vi "AlliGator Compute Valid Pixels Array.vi"(7 "Optional Rectangle":i32[](array[numeric]), 8 "error in (no error)":errorcluster, 10 "Pixel Counts Constraints":T1 {"High Count Pixels Rejection Options"."High Percentile" min=0.0 max=100.0; "Low Count Pixels Rejection Options"."Low Percentile" min=0.0 max=100.0}, 11 "Sum Image":T4) -> (0 "error out":errorcluster, 1 "CPU (s)":dbl, 2 "[[Valid Pixel (1,NaN)]] VxH Array":sgl[][](array[numeric]), 3 "[[Valid Pixel]] VxH Array":bool[][](array[boolean]), 4 "Message":string)   [LabVIEW 2021, in "AlliGator Phasor Plot.lvlib"]
doc: "Computes a boolean array specifying whether each pixel is valid (verifies all user-defined constraints)."
uses:
  AlliGator Phasor Plot.lvlib
  <vilib>/vision/Image Controls.llb/IMAQ Image.ctl
  AlliGator Pixel Counts Constraints.ctl
  AlliGator High Count Pixels Rejection Options.ctl
  AlliGator Low Count Pixels Rejection Options.ctl
  AlliGator Settings List.ctl
  <vilib>/vision/EDVR.llb/IMAQ ImageToEDVR 2D SGL.vi
  Variant/Variant to Data/Variant to Boolean.vi
  AlliGator Source Image.lvlib
  Arrays/Arrays.lvlib
  AlliGator ROIs.lvlib
  AlliGator Settings.lvlib
  Variant/Variant to Data/Variant to Data.lvlib
  <vilib>/vision/NI_Vision_Development_Module.lvlib
  Error/Error.lvlib
  Strings/Strings.lvlib
  Time/Time.lvlib
panel:
  out "# Valid Pixels":i32
  # "see the AlliGator License on the block diagram (Ctrl+E or Window:Show Block Diagram)"
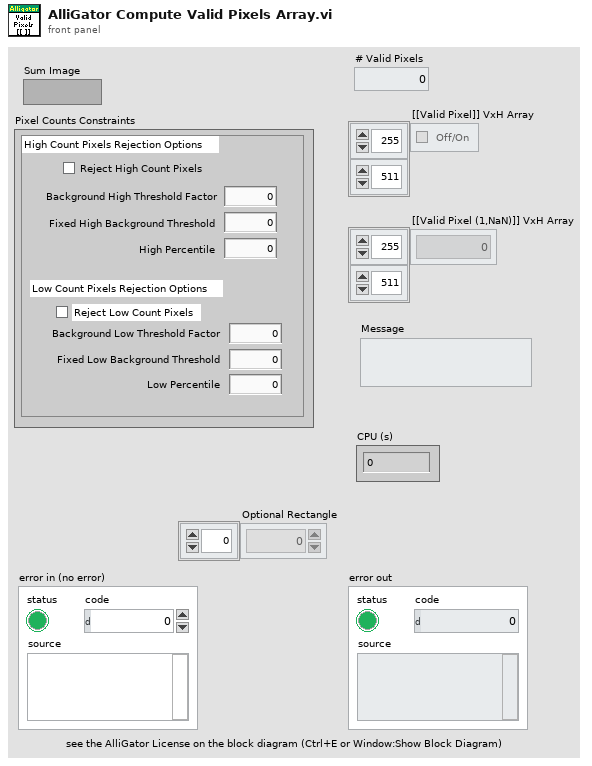
[diagram p1: front panel]
types:
  T1 = typedef "AlliGator Settings.lvlib/AlliGator Pixel Counts Constraints.ctl" = cluster{"High Count Pixels Rejection Options":T2, "Low Count Pixels Rejection Options":T3}
  T2 = typedef "AlliGator Settings.lvlib/AlliGator High Count Pixels Rejection Options.ctl" = cluster{"Background High Threshold Factor":dbl, "Fixed High Background Threshold":dbl, "Reject High Count Pixels":bool, "High Percentile":dbl}
  T3 = typedef "AlliGator Settings.lvlib/AlliGator Low Count Pixels Rejection Options.ctl" = cluster{"Background Low Threshold Factor":dbl, "Fixed Low Background Threshold":dbl, "Reject Low Count Pixels":bool, "Low Percentile":dbl}
  T4 = typedef "IMAQ Image.ctl" = refnum<image>
  T5 = typedef "AlliGator Settings.lvlib/AlliGator Settings List.ctl" = enum16{"GUI:Visible Settings Tab", "GUI:Last Run Version", "Source Image:Use Image Histogram for Contrast", "Source Image:Low Count Pixels Rejection Options", "Source Image:High Count Pixels Rejection Options", "Source Image:Use Image Brightness", "Source Image:Blend Overlay with Image Background", "Source Image:Use Fixed ROI Diameter", "Source Image:ROI Diameter", "Source Image:ROI Center Color", "Source Image:Peak Threshold", "Source Image:Intensity Threshold", "Source Image:Image Binning Options", "Source Image:Image Smoothing Options", "Source Image:Image Histogram Active", "Source Image:Invert Binary Mask", "Source Image:Hot Pixel Removal", "Source Image:Overlay Analyzed ROI Center", "Source Image:Auto-Adjust Contrast", "Source Image:Histogram Lower Percentile", "Source Image:Histogram Upper Percentile", "Source Image:Save Source Image", "Source Image:Scale Bar Options", "Source Image:Image Resolution (Pixel Size)", "Source Image:Flatfield Correction", "Source Image:Show Dead Left Columns Correction", "Source Image:Dead Left Columns Correction", "Source Image:Image Pre-Processing Operations Order", "Source Image:Overlay ROI Median", "Source Image:Median Overlay Color", "Data Information:Gate Width", "Data Information:Nanotime Gate Separation", "Data Information:Macrotime Gate Separation", "Data Information:Gate Step", "Data Information:# Gates", "Data Information:Gate Image Exposure", "Data Information:Gate Image Integration", "Data Information:Gates to Skip", "Data Information:Gates to Keep", "Data Information:Define Gates to", "Data Information:Channel Name", "Data Information:Available Channel Names", "Data Information:Channel Arithmetic", "Data Information:Background File Subtraction", "Data Information:Background File", "Data Information:Background Scaling Factor", "Data Information:Background Pile-up Correction", "Data Information:Background Pixel Well Capacity", "Data Information:Laser Period", "Data Information:SYNC Period", "Data Information:Pile-up Correction", "Data Information:Pixel Well Capacity", "Data Information:Dataset Scaling Factor", "Fluorescence Decay_Decay Pre-Processing:Reverse Gates", "Fluorescence Decay_Decay Pre-Processing:Verbose Decay Pre-Processing", "Fluorescence Decay_Decay Pre-Processing:Use Decay Pre-Processing", "Fluorescence Decay_Decay Pre-Processing:Background Subtraction", "Fluorescence Decay_Decay Pre-Processing:Background Definition Range", "Fluorescence Decay_Decay Pre-Processing:Baseline Subtraction Method", "Fluorescence Decay_Decay Pre-Processing:Decay Pre-Processing Operations Order", "Fluorescence Decay_Decay Pre-Processing:Smoothing Parameter", "Fluorescence Decay_Decay Pre-Processing:Shift Decay", "Fluorescence Decay_Decay Pre-Processing:Decay Shift Parameters", "Fluorescence Decay_Decay Pre-Processing:Fold Decay", "Fluorescence Decay_Decay Pre-Processing:# Folds", "Fluorescence Decay_Decay Pre-Processing:1-Normalize Decay", "Fluorescence Decay_Decay Pre-Processing:[0-1]-Normalize Decay", "Fluorescence Decay_Decay Pre-Processing:Smoothen Decay", "Fluorescence Decay_Decay Pre-Processing:Extrapolate Decay", "Fluorescence Decay_Decay Pre-Processing:Use Periodicity", "Fluorescence Decay_Decay Pre-Processing:Use Cursors", "Fluorescence Decay_Decay Pre-Processing:Tail Fraction", "Fluorescence Decay_Decay Pre-Processing:Head Fraction", "Fluorescence Decay_Decay Pre-Processing:Additional Points", "Fluorescence Decay_Decay Pre-Processing:Straighten Decay", "Fluorescence Decay_Decay Pre-Processing:Constant Background", "Fluorescence Decay_Decay Pre-Processing:Pixel-Normalize Decay", "Fluorescence Decay_Advanced Analysis:Extract IRF instead of Decay", "Fluorescence Decay_Advanced Analysis:IRF Extraction Options", "Fluorescence Decay_Advanced Analysis:IRF Optimization Options", "Fluorescence Decay_Advanced Analysis:Square Pulse Options", "Fluorescence Decay_Advanced Analysis:IRF Order", "Fluorescence Decay_Advanced Analysis:IRF Time Constants", "Fluorescence Decay_Advanced Analysis:Wavelet Analysis Options", "Fluorescence Decay_Advanced Analysis:Average Lifetime Options", "Fluorescence Decay_Fit Options:Fit Options", "Fluorescence Decay_Fit Options:Use Legacy Fitting Approach", "Fluorescence Decay_Fit Options:Use Data Information Laser Period", "Fluorescence Decay_Fit Parameters:Displayed Fit Parameters", "Fluorescence Decay_Fit Parameters:Fit Parameter Constraints", "Fluorescence Decay_Fit Parameters:Export Tabulated Results", "Fluorescence Decay_Fit Parameters:MLE Baseline Offset Type", "Fluorescence Decay_Fit Parameters:MLE Baseline Offset", "Fluorescence Decay_Fit Parameters:Guess Parameter Names", "Fluorescence Decay_Fit Parameters:Guess Parameter Values", "Fluorescence Decay_Fit Parameters:Guess Parameters Options", "Fluorescence Decay_Styles:Show Last Decay Only", "Fluorescence Decay_Styles:Decay Graph Color Array", "Fluorescence Decay:Decay Graph Active", "Fluorescence Decay Statistics:Min Peak Value", "Fluorescence Decay Statistics:Reject Low Decay Peak Pixels", "Fluorescence Decay Statistics:Reject High Decay Peak Pixels", "Fluorescence Decay Statistics:Max Peak Value", "Time Traces:Use File Timestamp", "Time Traces:Time Step", "Time Traces:Use Intensity Correction File", "Time Traces:Intensity Correction File", "Phasor Plot:Phasor Plot Smoothing Options", "Phasor Plot:Phasor Plot Size", "Phasor Plot:Phasor Plot Graphics Options", "Phasor Plot:Cumulative Phasor Plot", "Phasor Plot:Use Phasor Brightness", "Phasor Plot:Blend Overlay with Phasor Background", "Phasor Plot:Save Phasor Plot", "Phasor Plot:Show References", "Phasor Plot:Phasor Ratio Decay Range", "Phasor Plot:Exponential Fading", "Phasor Plot:Phasor Ratio Reference Colors", "Phasor Plot:Reference Radius", "Phasor Plot:Show Color Map Vertices", "Phasor Plot:Phasor Plot Active", "Phasor Plot:Phasor Ratio Color Map Type", "Phasor Plot:Phasor Ratio Color Map", "Phasor Plot:Phasor Ratio Display Range", "Phasor Plot:Selected Image ROI(s)", "Phasor Plot:All Image ROIs", "Phasor Plot:Selected Phasor Plot ROI(s)", "Phasor Plot:All Phasor Plot ROIs", "Phasor Plot:Phasor Ratio Color-Coded Quantity", "Phasor Plot:Store Phasor Harmonics", "Phasor Plot:Draw Reference Segment", "Phasor Plot:User-Defined Quantity", "Phasor Graph:Phasor Frequency", "Phasor Graph:Phasor Ratio Type", "Phasor Graph:Pixel-level Phasor Computation", "Phasor Graph:Save Phasor Graph", "Phasor Graph:Phasor Graph Active", "Phasor Graph:Phasor SDV Options", "Phasor Calibration:Use Backup Calibration if needed", "Phasor Graph:Define Shortest Lifetime as", "Phasor Calibration:Backup Calibration Type", "Phasor Calibration:Calibration Type", "Phasor Calibration:Calibration Lifetime", "Phasor Calibration:Calibration Map Algorithm", "Single-Exponential Phasor Locus (SEPL):Gate Parameters", "Single-Exponential Phasor Locus (SEPL):User-defined Gate", "Single-Exponential Phasor Locus (SEPL):User-defined IRF", "Single-Exponential Phasor Locus (SEPL):Phasor Parameters", "Single-Exponential Phasor Locus (SEPL):Decay & IRF Parameters", "Single-Exponential Phasor Locus (SEPL):Display Parameters", "Lifetime Analysis:Decay Analysis Parameters", "Lifetime Analysis:Lifetime Map Active", "Plugins:Python Settings", "Miscellaneous:Verbose Mode", "Miscellaneous:Beep after Script", "Miscellaneous:Saved Image File Format", "Miscellaneous:Exported Gate Image Settings", "Miscellaneous:Include Loading in Timing", "Miscellaneous:Verbose Settings Mode", "Miscellaneous:Histogram Options", "Miscellaneous:Beep on Error", "Miscellaneous:# Logical Processors Used", "Miscellaneous:ROI Description Max Characters", "Miscellaneous:Verbose Error Mode", "Miscellaneous:Transparent Mask Color"}
  T6 = typedef "Image Type" = u32
  T7 = typedef "Image.lvlib/Named ROI Description.ctl" = cluster{"ROI Descriptor":T8, "ROI Name":string, "Overlay Color":u32}
  T8 = typedef "ROI Descriptor" = cluster{"Global Rectangle":i32[], "Contours":cluster{"ID":enum32{"External", "Internal"}, "Type":u32, "Coordinates":i32[]}[]}
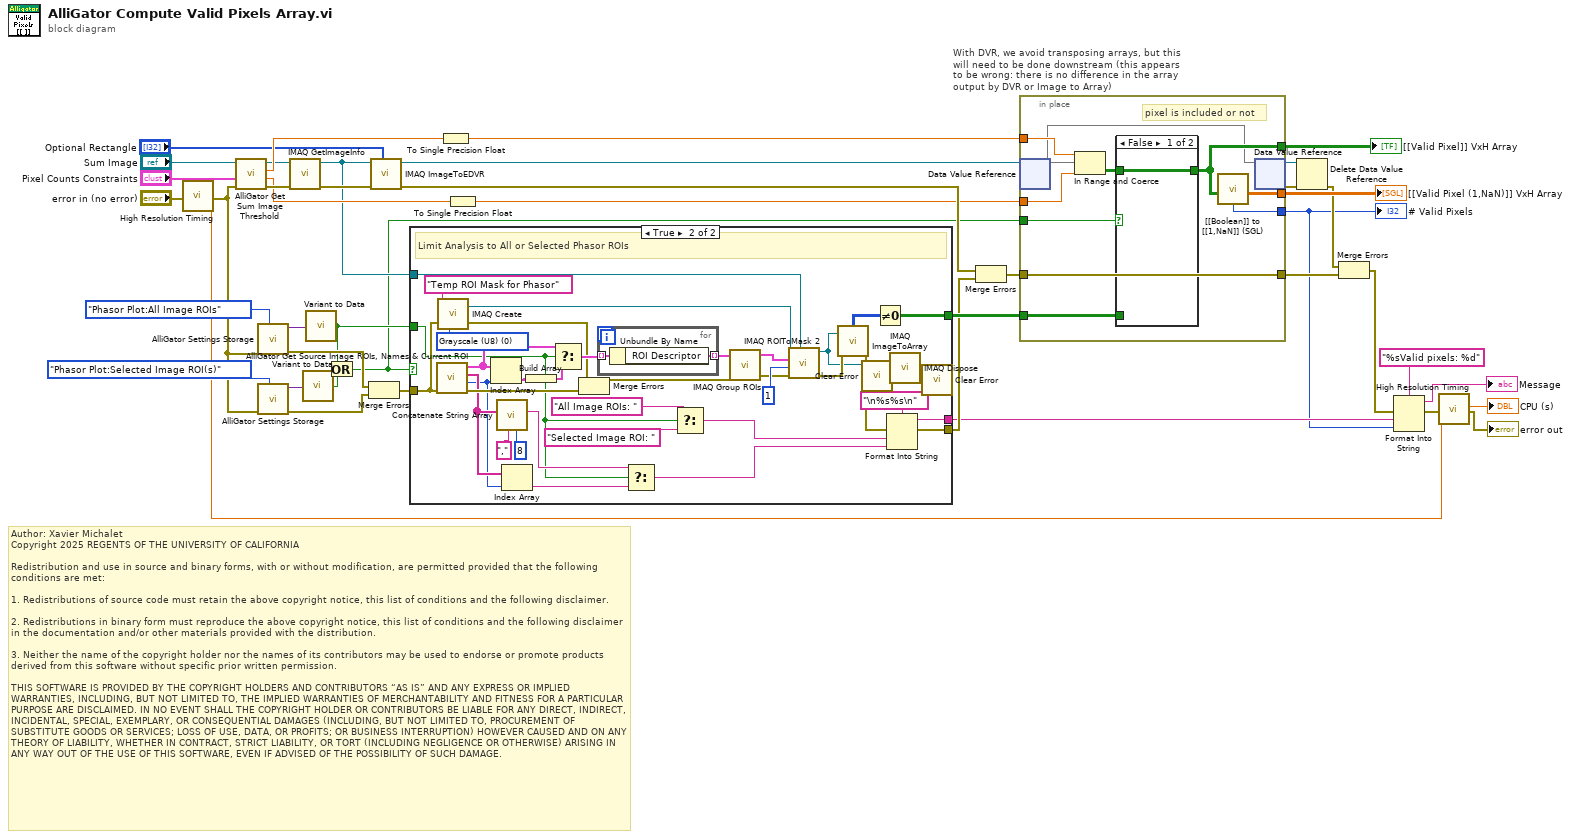
[diagram p0: block diagram]
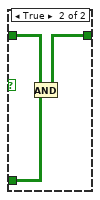
[diagram p2: hidden frame]
diagram:
  # "Author: Xavier Michalet\nCopyright 2025 REGENTS OF THE UNIVERSITY OF CALIFORNIA\n\nRedistribution and use in source and binary forms, with or without modification, are permitted provided that the following conditions are met:\n\n1. Redistributions of source code must retain the above copyright notice, this list of conditions and the following disclaimer.\n\n2. Redistributions in binary form must reproduce the above copyright notice, this list of conditions and the following disclaimer in the documentation and/or other materials provided with the distribution.\n\n3. Neither the name of the copyright holder nor the names of its contributors may be used to endorse or promote products derived from this software without specific prior written permission.\n\nTHIS SOFTWARE IS PROVIDED BY THE COPYRIGHT HOLDERS AND CONTRIBUTORS “AS IS” AND ANY EXPRESS OR IMPLIED WARRANTIES, INCLUDING, BUT NOT LIMITED TO, THE IMPLIED WARRANTIES OF MERCHANTABILITY AND FITNESS FOR A PARTICULAR PURPOSE ARE DISCLAIMED. IN NO EVENT SHALL THE COPYRIGHT HOLDER OR CONTRIBUTORS BE LIABLE FOR ANY DIRECT, INDIRECT, INCIDENTAL, SPECIAL, EXEMPLARY, OR CONSEQUENTIAL DAMAGES (INCLUDING, BUT NOT LIMITED TO, PROCUREMENT OF SUBSTITUTE GOODS OR SERVICES; LOSS OF USE, DATA, OR PROFITS; OR BUSINESS INTERRUPTION) HOWEVER CAUSED AND ON ANY THEORY OF LIABILITY, WHETHER IN CONTRACT, STRICT LIABILITY, OR TORT (INCLUDING NEGLIGENCE OR OTHERWISE) ARISING IN ANY WAY OUT OF THE USE OF THIS SOFTWARE, EVEN IF ADVISED OF THE POSSIBILITY OF SUCH DAMAGE."
  n1 = call "High Resolution Timing.vi"("Error In"="error in (no error)") -> ("elapsed (relative) seconds"=w2:dbl, "Error Out"=w4:errorcluster)  [unwired: 16 in, 1 out]
  n2 = call "AlliGator Get Sum Image Threshold.vi"("error in (no error)"=w4, "Pixel Counts Constraints"="Pixel Counts Constraints", "Image in"="Sum Image") -> ("error out"=w41:errorcluster, "Pixel Threshold Low"=w39:sgl, "Pixel Threshold High"=w40:sgl, "Image out (dup)"=w15:T4)  [unwired: 2 in, 3 out]
  n3 = call "AlliGator Settings Storage.vi"("AlliGator Settings List"=AlliGator_Settings_List."Phasor Plot:All Image ROIs", "Error In"=w4) -> ("Error Out"=w19:errorcluster, "Variant Data out"=w22:variant)  [unwired: 8 in]
  n4 = call "AlliGator Settings Storage.vi"("AlliGator Settings List"=AlliGator_Settings_List."Phasor Plot:Selected Image ROI(s)", "Error In"=w4) -> ("Error Out"=w18:errorcluster, "Variant Data out"=w21:variant)  [unwired: 8 in]
  n5 = call "IMAQ GetImageInfo"("error in (no error)"=w41, "Image"=w15) -> ("error out"=w42:errorcluster)  [unwired: 2 in, 7 out]
  n6 = call-poly "Variant to Data.vi"("Variant"=w21) -> ("Value"=w20:bool)  [unwired: 8 in]
  n7 = call-poly "Variant to Data.vi"("Variant"=w22) -> ("Value"=w16:bool)  [unwired: 8 in]
  n8 = Or(x=w16, y=w20) -> (x .or. y?=w13:bool)
  n9 = Merge Errors(w19, w18) -> (w17:errorcluster)
  n10 = call-poly <vilib>:"IMAQ ImageToEDVR.vi"("Optional Rectangle"="Optional Rectangle", "error in (no error)"=w42, "Image"=w15) -> ("error out"=w31:errorcluster, "EDVR 2D SGL"=w30:refnum<data-value>)  [unwired: 6 in, 1 out]
  n11 = case shown="True" w13 {
    tunnel: w17 -> [w43 w74]
    tunnel: w16 -> [_ w53]
    tunnel: w15 -> [_ w69]
    tunnel: [_ w71] -> w14
    tunnel: [w43 w47] -> w8
    tunnel: [_ w46] -> w7
    frame False {
    }
    frame True {
      w72 = T6 0 items=["Grayscale (U8)", "Grayscale (I16)", "Grayscale (SGL)", "Complex (CSG)", "RGB (U32)", "HSL (U32)", "RGB (U64)", "Grayscale (U16)"] ("Image Type")
      # "Limit Analysis to All or Selected Phasor ROIs"
      n12 = call "AlliGator Get Source Image ROIs, Names & Current ROI.vi"("Error In"=w74) -> ("Error Out"=w76:errorcluster, "Current ROI"=w55:i32, "ROI Names"=w57:string[], "Stored ROIs"=w80:T7[])  [unwired: 7 in]
      n13 = call "IMAQ Create"("Image Name"="Temp ROI Mask for Phasor", "Image Type"=w72, "error in (no error)"=w74) -> ("New Image"=w68:T4, "error out"=w73:errorcluster)  [unwired: 2 in]
      n14 = Index Array(array=w80, index=w55) -> (element=w79:T7)
      n15 = call "Concatenate String Array.vi"("Max Number of Elements (None: -1)"=8, "Separator (TAB)"=",", "String Array"=w57) -> ("Formatted String"=w56:string)  [unwired: 8 in]
      n16 = Index Array(array=w57, index=w55) -> (element=w54:string)
      n17 = Build Array(w79) -> (w78:T7[])
      n18 = Select(t=w80, s=w53, f=w78) -> (s? t:f=w77:T7[])
      n19 = Merge Errors(w73, w76) -> (w63:errorcluster)
      n20 = for {
        tunnel: w77 -> [w82] mode=indexing
        tunnel: [w81] -> w64 mode=indexing
        n21 = Unbundle By Name(w82) -> ("ROI Descriptor"=w81:T8)
      }
      n22 = Select(t=w56, s=w53, f=w54) -> (s? t:f=w49:string)
      n23 = Select(t="All Image ROIs: " ("Prefix (\"\")"), s=w53, f="Selected Image ROI: ") -> (s? t:f=w50:string)
      n24 = call "IMAQ Group ROIs"("error in (no error)"=w63, "ROI Descriptors"=w64) -> ("error out"=w61:errorcluster, "ROI Descriptor out"=w62:T8)  [unwired: 2 in]
      n25 = call "IMAQ ROIToMask 2"("Image Model"=w69, "error in (no error)"=w61, "Filling Value (255)"=1, "ROI Descriptor"=w62, "Image"=w68) -> ("error out"=w67:errorcluster, "Image Out"=w66:T4)  [unwired: 4 in, 1 out]
      n26 = call "IMAQ ImageToArray"("error in (no error)"=w67, "Image"=w66) -> ("error out"=w48:errorcluster, "Image Pixels (U8)"=w70:u8[][])  [unwired: 2 in, 3 out]
      n27 = call "Clear Error.vi"("Error In"=w48) -> ("no Error Out"=w44:errorcluster)  [unwired: 8 in]
      n28 = Not Equal To 0?(x=w70) -> (x != 0?=w71:bool[][])
      n29 = Format Into String(format string="\n%s%s\n", error in=w48, w50, w49) -> (resulting string=w46:string, error out=w47:errorcluster)  [unwired: 1 in]
      n30 = call "IMAQ Dispose"("Image"=w66, "error in (no error)"=w44) -> ("error out"=w60:errorcluster)  [unwired: 4 in]
      n31 = call "Clear Error.vi"("Error In"=w60) -> ()  [unwired: 8 in, 1 out]
    }
  }
  n32 = To Single Precision Float(number=w40) -> (single precision float=w34:sgl)
  n33 = To Single Precision Float(number=w39) -> (single precision float=w28:sgl)
  n34 = Merge Errors(w31, w8) -> (w9:errorcluster)
  n35 = in-place "With DVR, we avoid transposing arrays, but this will need to be done downstream (this appears to be wrong: there is no difference in the array output by DVR or Image to Array)" {
    in-place-border: w28 -> [w90]
    in-place-border: [w89] -> w35
    in-place-border: w9 -> [w92]
    in-place-border: [w92] -> w29
    in-place-border: w34 -> [w91]
    in-place-border: [w84] -> w36
    in-place-border: [w88] -> w5
    in-place-border: w14 -> [w85]
    in-place-border: w13 -> [w87]
    # "pixel is included or not"
    n36 = in-place-dvr #1(w30) -> (w83:sgl[][])  [unwired: 1 out]
    n37 = In Range and Coerce(upper limit=w91, x=w83, lower limit=w90) -> (In Range?=w86:bool[][])  [unwired: 1 out]
    n38 = case shown="False" w87 {
      tunnel: w86 -> [w93 w96]
      tunnel: w85 -> [_ w95]
      tunnel: [w93 w94] -> w84
      frame False {
      }
      frame True {
        n39 = And(x=w96, y=w95) -> (x .and. y?=w94:bool[][])
      }
    }
    n40 = call "[[Boolean]] to [[1,NaN]] (SGL).vi"("Valid?"=w84) -> ("# Valid"=w88:i32, "1 or NaN Array"=w89:sgl[][])  [unwired: 3 in]
    n41 = in-place-dvr #1(w83) -> (w32:refnum<data-value>, w33:errorcluster)
  }
  "[[Valid Pixel]] VxH Array" <- w36
  "[[Valid Pixel (1,NaN)]] VxH Array" <- w35
  "# Valid Pixels" <- w5
  n42 = Delete Data Value Reference(data value reference=w32, error in=w33) -> (error out=w26:errorcluster)  [unwired: 1 out]
  n43 = Merge Errors(w26, w29) -> (w11:errorcluster)
  n44 = Format Into String(format string="%sValid pixels: %d", error in=w11, w7, w5) -> (resulting string=→"Message":string, error out=w10:errorcluster)  [unwired: 1 in]
  n45 = call "High Resolution Timing.vi"("relative seconds (NaN)"=w2, "Error In"=w10) -> ("elapsed (relative) seconds"=→"CPU (s)":dbl, "Error Out"=→"error out":errorcluster)  [unwired: 15 in, 1 out]
